vi "Test_Glob_1.vi"() -> ()   [LabVIEW 2020]
uses:
  Modules/Fonction Standard/Fichier ou dossier/Cluster des Chemins.ctl
panel:
  in  "Quitter":bool
  in  "Output VISA Imprimante":refnum<visa-resource-name>="TCPIP0::10.41.9.129::9100::socket"
  out "Numéro scanné":string
  in  "Carton Numéro":i16=1
  in  "nom VISA Lecteur code barre":refnum<visa-resource-name>="COM1"
  in  "DATA cmde":T1={"n°article FAS"="12-216C-04521 EQIFIL 417mA 14.4ohm", "n° cmde FAS"="03838/08-01.07.01", "quantité cmde"="100", "ID LIG cmde"="966584", "n° cmde client"="CF-08-0253/2", "nom client"="EMS Electro Medical System", "n° article client"="EL-360", "indice revision client"="03", "société de facturation"="FAS Medic", "langue a utiliser"="FR"}
  in  "N° carton":u8=1
  in  "Nb pièces par carton":u8=5
  in  "Tableau n° valves":string[](array[string])=["112105740008010001", "112105740008010002", "112105740008010003", "112105740008010004", "112105740008010005", "112105740008010006", "112105740008010007", "112105740008010008", "112105740008010009", "112105740008010010", "112105740008010011", "112105740008010012", "112105740008010013", "112105740008010014", "112105740008010015", "112105740008010016", "112105740008010017", "112105740008010018", "112105740008010019", "112105740008010020", "112105740008010021", "112105740008010022", "112105740008010023", "112105740008010024", "112105740008010025", "112105740008010026", "112105740008010027", "112105740008010028", "112105740008010029", "112105740008010030", "112105740008010031", "112105740008010032", "112105740008010033", "112105740008010034", "112105740008010035", "112105740008010036", "112105740008010037", "112105740008010038", "112105740008010039", "112105740008010040", "112105740008010041", "112105740008010042", "112105740008010043", "112105740008010044", "112105740008010045", "112105740008010046", "112105740008010047", "112105740008010048", "112105740008010049", "112105740008010050"]
  out "error out":errorcluster caption="sortie d'erreur"
  out "n° lot à scanner":string
  in  "Tableau \nlots OUT":string[][](array[string])
  in  "Chemins":T2={" Admin-réseau "=path "\\\\Plz-inf-nas\\medic/PARAMETRES_TESTS/PROD_Data-Admin", " XML-Réseau"=path "\\\\Plz-inf-nas\\medic/PARAMETRES_TESTS/FlatpropConfig", " Résultat tests-Réseau"=path "\\\\Plz-inf-nas\\medic/FASMedic_Methodes_MTD/TRACABILITE", " Archive prôbleme-Réseau"=path "\\\\Plz-inf-nas\\Medic/RELEVES AUTOMATIQUES/Archives probleme reseau", " Archive Test  Local"=path "C:/Archive Test"}
  in  "entrée d'erreur":errorcluster
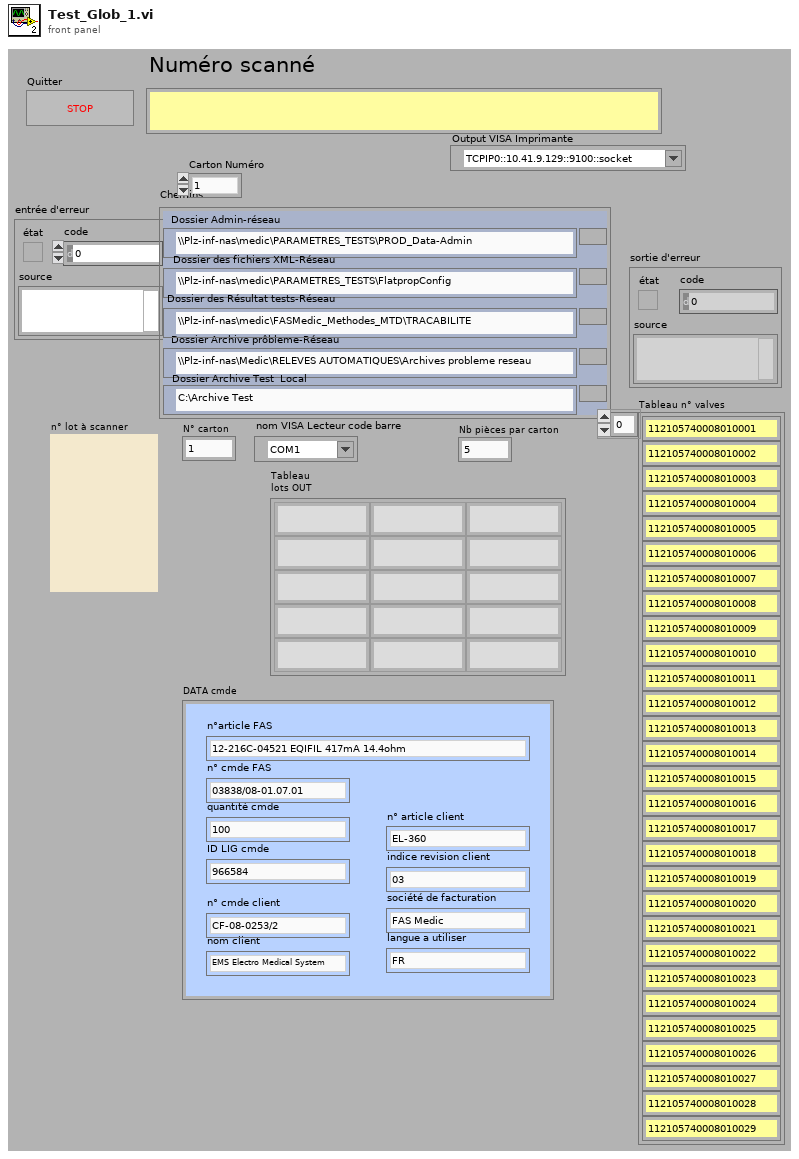
[diagram p1: front panel]
types:
  T1 = typedef "DATA commande.ctl" = cluster{"n°article FAS":string, "n° cmde FAS":string, "quantité cmde":string, "ID LIG cmde":string, "n° cmde client":string, "nom client":string, "n° article client":string, "indice revision client":string, "société de facturation":string, "langue a utiliser":string}
  T2 = typedef "Cluster des Chemins.ctl" = cluster{" Admin-réseau ":path, " XML-Réseau":path, " Résultat tests-Réseau":path, " Archive prôbleme-Réseau":path, " Archive Test  Local":path}
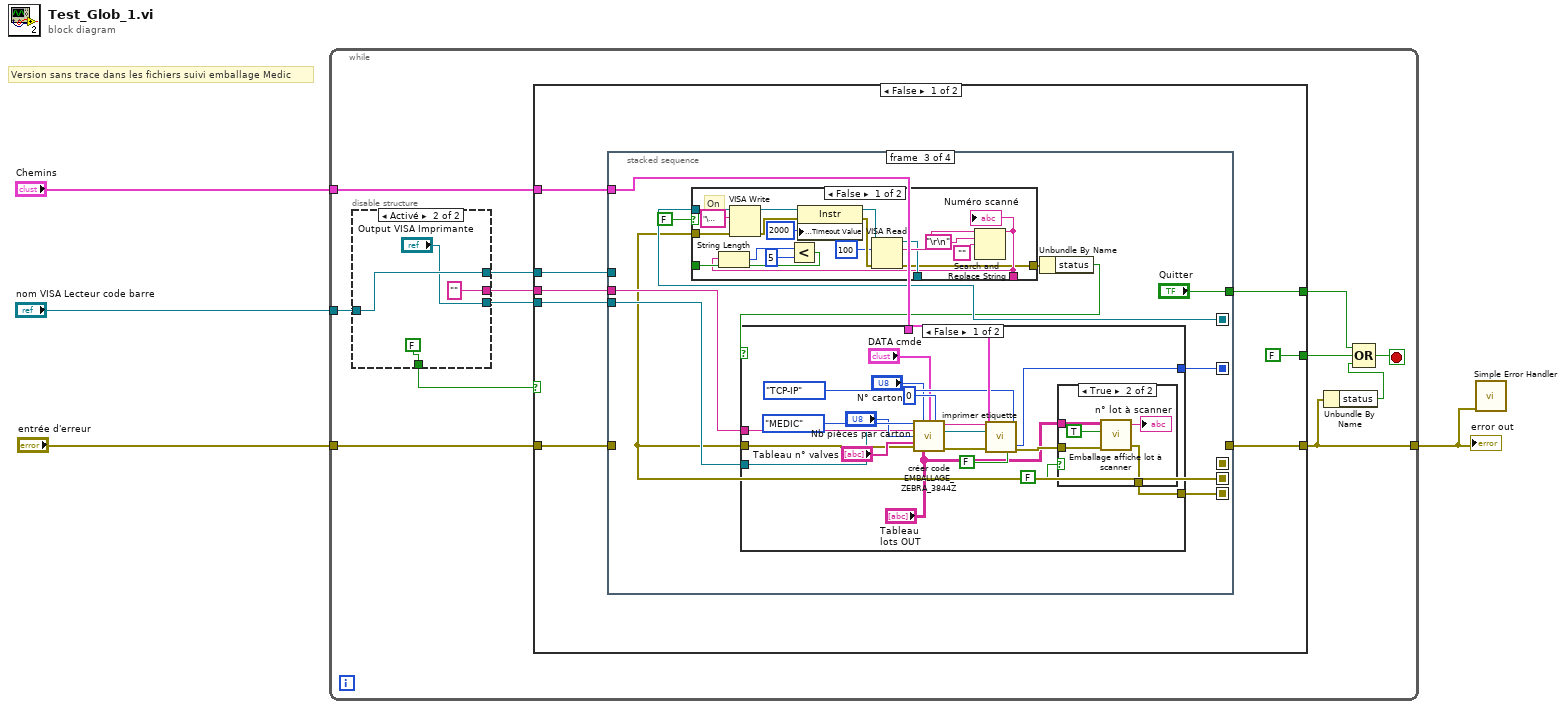
[diagram p0: block diagram]
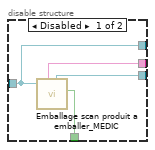
[diagram p2: hidden frame]
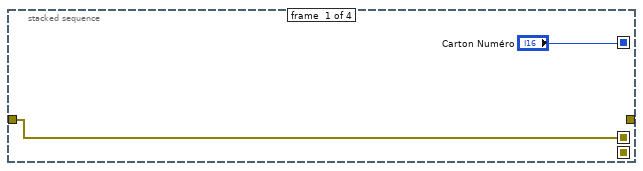
[diagram p3: hidden frame]
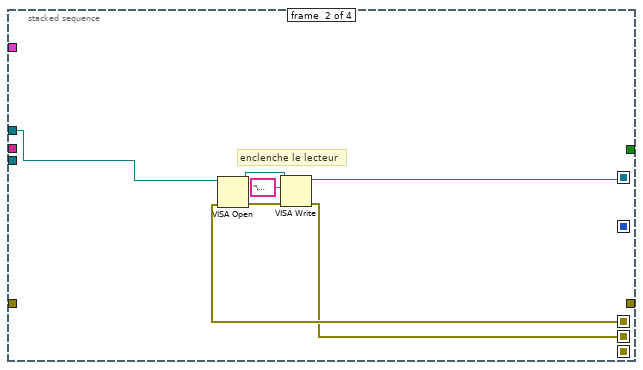
[diagram p4: hidden frame]
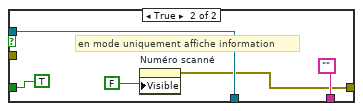
[diagram p7: hidden frame]
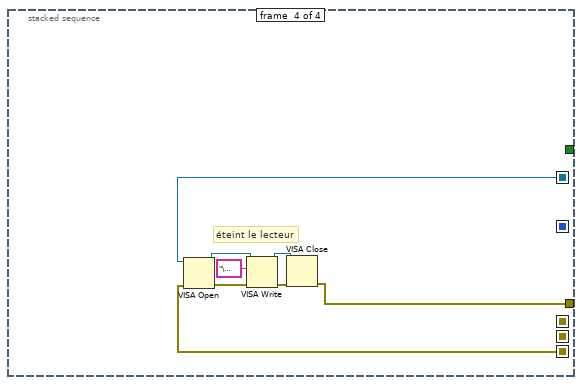
[diagram p8: hidden frame]
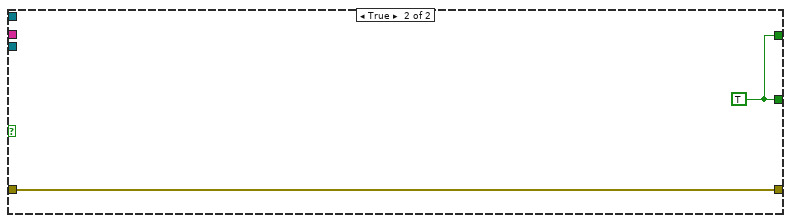
[diagram p9: hidden frame]
diagram:
  # "Version sans trace dans les fichiers suivi emballage Medic"
  n1 = while {
    tunnel: "Chemins" -> [w16]
    tunnel: "nom VISA Lecteur code barre" -> [w14]
    tunnel: "entrée d'erreur" -> [w13]
    tunnel: [w10] -> w1
    stop <- w11 stop-if-true
    n2 = disable-structure shown="Activé" {
      disable-tunnel: [w20 "Output VISA Imprimante"] -> w15
      disable-tunnel: w14 -> [w17 w22]
      disable-tunnel: [w19 FALSE ("Arrêter le programme (T)")] -> w9
      disable-tunnel: [w18 "" ("Nom du produit")] -> w7
      disable-tunnel: [w17 w22] -> w6
      frame Disabled {
        n3 = call "Emballage scan produit a emballer_MEDIC.vi"("nom de ressource VISA"=w17) -> ("Nom du produit"=w18:string, "Output VISA Imprimante"=w20:refnum<visa-resource-name>, "Arrêter le programme (T)"=w19:bool)  [unwired: 3 in, 4 out]
      }
      frame Enabled {
      }
    }
    n4 = case shown="False" w9 {
      tunnel: w16 -> [w32 _]
      tunnel: w15 -> [w31 _]
      tunnel: w13 -> [w30 w111]
      tunnel: [w29 w111] -> w10
      tunnel: [FALSE w110] -> w8
      tunnel: w7 -> [w27 _]
      tunnel: w6 -> [w26 _]
      tunnel: [w25 w110] -> w5
      frame False {
        n5 = stacked-sequence {
          seq-local: ["Carton Numéro" _ _ _] -> [_ _ w50 _]
          seq-local: [_ w38 _ _] -> [_ _ w47 w104]
          seq-local: [w33 _ _ _] -> [_ w37 _ _]
          seq-local: [_ w36 _ _] -> [_ _ w46 _]
          seq-local: [_ _ w48 _] -> [_ _ _ w103]
          tunnel: w32 -> [_ _ w52 _]
          tunnel: w31 -> [_ _ w51 _]
          tunnel: w30 -> [w33 _ _ _]
          tunnel: [_ _ _ w102] -> w29
          tunnel: w27 -> [_ _ w49 _]
          tunnel: w26 -> [_ w35 _ _]
          tunnel: [_ _ "Quitter" _] -> w25
          frame #0 {
          }
          frame #1 {
            # "enclenche le lecteur"
            n6 = VISA Open(error in (no error)=w37, VISA resource name=w35) -> (VISA resource name=w39:refnum<visa-resource-name>, error out=w40:errorcluster)  [unwired: 3 in]
            n7 = VISA Write(VISA resource name=w39, write buffer="\u0002", error in (no error)=w40) -> (VISA resource name out=w38:refnum<visa-resource-name>, error out=w36:errorcluster)  [unwired: 1 out]
          }
          frame #2 {
            n8 = case shown="False" FALSE {
              tunnel: w47 -> [w87 w100]
              tunnel: [w85 TRUE] -> _
              tunnel: [w84 w100] -> _
              tunnel: [w83 ""] -> _
              tunnel: w46 -> [w82 _]
              tunnel: [w81 w97] -> w45
              frame False {
                # "On"
                n9 = VISA Write(VISA resource name=w87, write buffer="\u0002", error in (no error)=w82) -> (VISA resource name out=w88:refnum<visa-resource-name>, error out=w89:errorcluster)  [unwired: 1 out]
                n10 = property class="Instr"(reference=w88, error in=w89, "General Settings:Timeout Value"=u32 2000 ("Tmo Value")) -> (reference out=w95:refnum<visa-resource-name>, error out=w96:errorcluster)
                n11 = VISA Read(VISA resource name=w95, byte count=u32 100 ("byte count (0)"), error in (no error)=w96) -> (VISA resource name out=w84:refnum<visa-resource-name>, read buffer=w92:string, error out=w81:errorcluster)  [unwired: 1 out]
                n12 = Search and Replace String(input string=w92, search string="\r\n", replace string="") -> (result string=w83:string)  [unwired: 5 in, 3 out]
                "Numéro scanné" <- w83
                n13 = String Length(string=w83) -> (length=w80:i32)
                n14 = Less?(x=w80, y=5) -> (x < y?=w85:bool)
              }
              frame True {
                # "en mode uniquement affiche information"
                n15 = property on="Numéro scanné" class="Str"("Visible"=FALSE) -> (error out=w97:errorcluster)  [unwired: 2 in, 1 out]
              }
            }
            n16 = Unbundle By Name(w45) -> ("status"=w44:bool)
            n17 = case shown="False" w44 {
              tunnel: w52 -> [w71 _]
              tunnel: w51 -> [w54 _]
              tunnel: w50 -> [w58 _]
              tunnel: w49 -> [w57 _]
              tunnel: [w56 w78] -> w48
              tunnel: w46 -> [w55 w78]
              frame False {
                n18 = call "créer code EMBALLAGE_ZEBRA_3844Z.vi"("DIVISION"=enum16{"FLATPROP", "MEDIC"}."MEDIC", "N° carton"="N° carton", "DATA cmde"="DATA cmde", "Nb total cartons"=0, 5:w57, 7:"Nb pièces par carton", "Tableau n° valves"="Tableau n° valves", "error in (no error)"=w55, "Tableau \nlots OUT"="Tableau \nlots OUT") -> ("chaine  à écrire"=w69:string, "error out"=w68:errorcluster)  [unwired: 3 in, 2 out]
                n19 = call "imprimer etiquette.vi"("chaine à écrire"=w69, "Type de liaison"=enum16{"RS232", "USB", "TCP-IP", "Aucune"}."TCP-IP", 5:w54, "sélecteur"=w71, "error in"=w68, "Carton Numéro"=w58, "fin de série ?"=FALSE) -> ("error out"=w67:errorcluster)  [unwired: 8 in]
                n20 = case shown="True" FALSE {
                  tunnel: w67 -> [w72 w77]
                  tunnel: "Tableau \nlots OUT" -> [_ w76]
                  tunnel: [w72 w73] -> w56
                  frame False {
                  }
                  frame True {
                    n21 = call "Emballage affiche lot à scanner.vi"("Tableau \nlots OUT"=w76, "Affiche ?"=TRUE, "error in (no error)"=w77) -> ("n° lot à scanner"=→"n° lot à scanner":string, "error out"=w73:errorcluster)  [unwired: 2 in, 1 out]
                  }
                }
              }
              frame True {
              }
            }
          }
          frame #3 {
            # "éteint le lecteur"
            n22 = VISA Open(error in (no error)=w103, VISA resource name=w104) -> (VISA resource name=w108:refnum<visa-resource-name>, error out=w106:errorcluster)  [unwired: 3 in]
            n23 = VISA Write(VISA resource name=w108, write buffer="\u0003", error in (no error)=w106) -> (VISA resource name out=w109:refnum<visa-resource-name>, error out=w107:errorcluster)  [unwired: 1 out]
            n24 = VISA Close(VISA resource name=w109, error in (no error)=w107) -> (error out=w102:errorcluster)
          }
        }
      }
      frame True {
        w110 = TRUE
      }
    }
    n25 = Unbundle By Name(w10) -> ("status"=w12:bool)
    n26 = Compound Arithmetic op=OR(w5, w8, w12) -> (w11:bool)
  }
  "error out" <- w1
  n27 = call <vilib>:"Simple Error Handler.vi"("error in (no error)"=w1) -> ()  [unwired: 4 in, 5 out]
